vi "Function_Flow Mark.vi"(8 "Error in":errorcluster, 9 "CoordSys In":T1 {"Measurement System"."Axis Reference" items=["Direct", "Indirect"]; "Measurement System"."Angle (deg)" format="%.2f"; "Measurement System"."Origin"."Y" format="%.2f"; "Measurement System"."Origin"."X" format="%.2f"; "Reference System"."Axis Reference" items=["Direct", "Indirect"]; "Reference System"."Angle (deg)" format="%.2f"; "Reference System"."Origin"."Y" format="%.2f"; "Reference System"."Origin"."X" format="%.2f"}, 10 "Data Cluster In":cluster{"Name":string, "Variant In":variant}, 11 "Image Dst In":T4) -> (0 "Error out":errorcluster, 1 "ROI Out":T2 {"Contours"."Type" items=["No Selection", "Point", "Line", "Rectangle", "Oval", "Polygon", "Free", "Annulus", "Unused2", "Unused3", "Broken Line", "Free Hand Line", "Rotated Rectangle"]}, 2 "Result(Flow Mark)":cluster{"Name":string, "NG?":bool, "Score":dbl}, 3 "Objects":T3(array[cluster]) {"Area" format="%.2f"; "Object Center"."Y" format="%.2f"; "Object Center"."X" format="%.2f"}, 4 "Time":u32)   [LabVIEW 2013]
uses:
  <vilib>/vision/Image Controls.llb/IMAQ Image.ctl
  Control/Control_Flow Mark.ctl
  <vilib>/vision/NI_Vision_Development_Module.lvlib
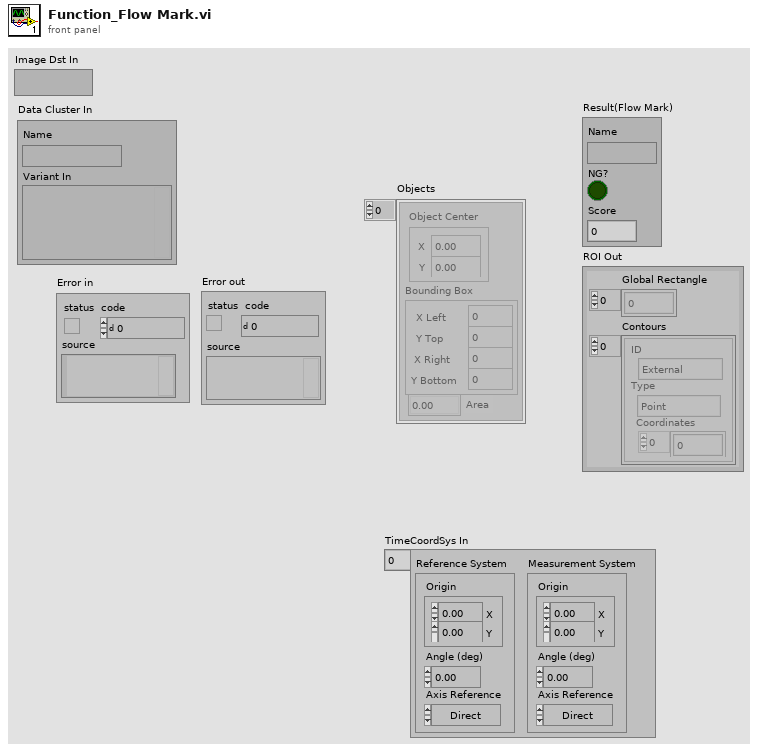
[diagram p1: front panel]
types:
  T1 = typedef "IMAQ Coordinate System" = cluster{"Reference System":cluster{"Origin":cluster{"X":sgl, "Y":sgl}, "Angle (deg)":sgl, "Axis Reference":u32}, "Measurement System":cluster{"Origin":cluster{"X":sgl, "Y":sgl}, "Angle (deg)":sgl, "Axis Reference":u32}}
  T2 = cluster{"Global Rectangle":i32[], "Contours":cluster{"ID":enum32{"External", "Internal"}, "Type":u32, "Coordinates":i32[]}[]}
  T3 = cluster{"Object Center":cluster{"X":dbl, "Y":dbl}, "Bounding Box":cluster{"X Left":dbl, "Y Top":dbl, "X Right":dbl, "Y Bottom":dbl}, "Area":dbl}[]
  T4 = typedef "IMAQ Image.ctl" = refnum<image>
  T5 = typedef "Control_Flow Mark.ctl" = cluster{"Name":string, "ROI":cluster{"Global Rectangle":i32[], "Contours":cluster{"ID":enum32{"External", "Internal"}, "Type":u32, "Coordinates":i32[]}[]}, "Extract Direction(¬y²ª)":enum16{"Left up", "Right up", "Left Down", "Right Down"}, "Extract Potion(¬y²ª)":cluster{"X":i32, "Y":i32}, "Magnification(¬y²ª)":i32, "Settings(¬y²ª)":cluster{"Objects":enum16{"Bright Objects", "Dark Objects"}, "Threshold":i32, "Min Object Size":bool, "Min Size":i32, "Max Object Size":bool, "Max Size":i32}}
  T6 = cluster{"Origin":cluster{"X":sgl, "Y":sgl}, "Angle (deg)":sgl, "Axis Reference":u32}
  T7 = enum16{"Left up", "Right up", "Left Down", "Right Down"}
  T8 = cluster{"Objects":enum16{"Bright Objects", "Dark Objects"}, "Threshold":i32, "Min Object Size":bool, "Min Size":i32, "Max Object Size":bool, "Max Size":i32}
  T9 = typedef "ROI Descriptor" = cluster{"Global Rectangle":i32[], "Contours":cluster{"ID":enum32{"External", "Internal"}, "Type":u32, "Coordinates":i32[]}[]}
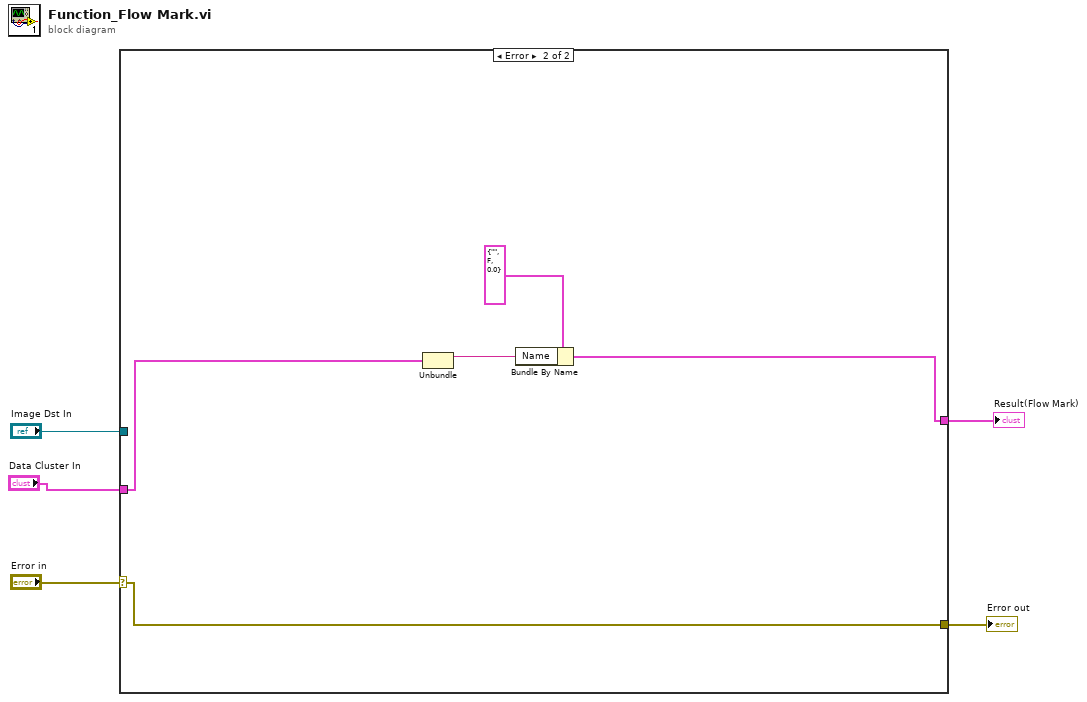
[diagram p0: block diagram]
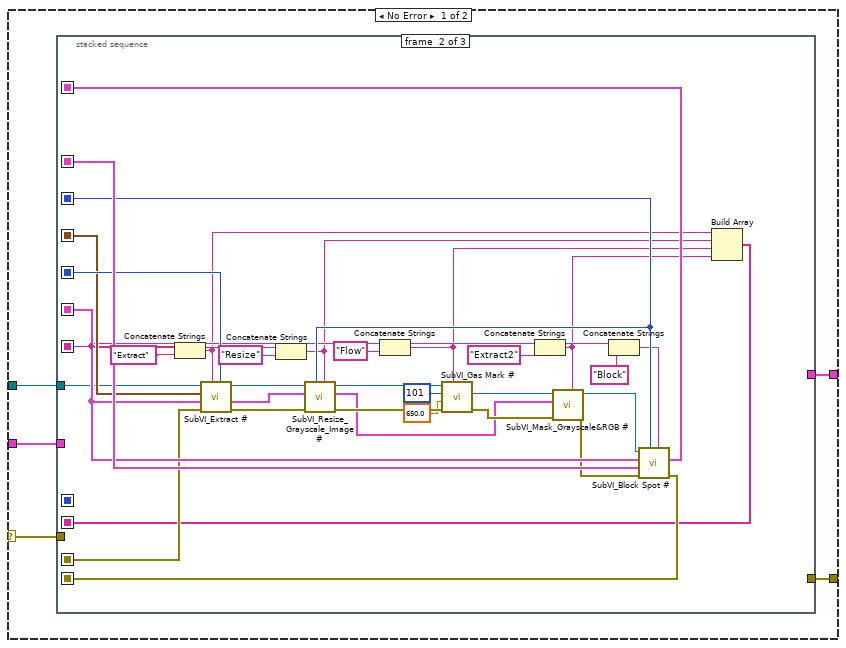
[diagram p2: hidden frame]
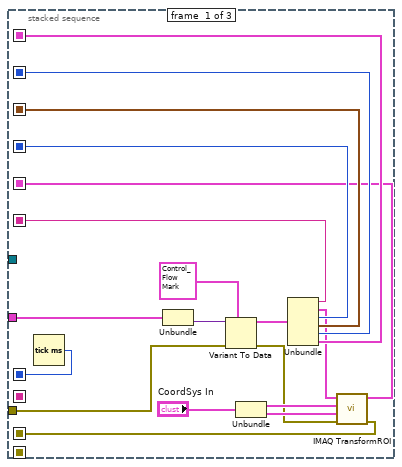
[diagram p3: hidden frame]
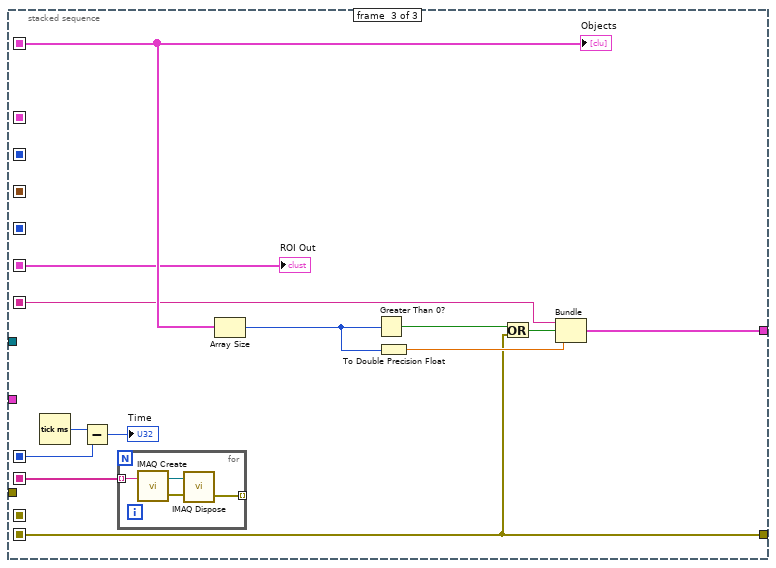
[diagram p4: hidden frame]
diagram:
  n1 = case shown="Error" "Error in" {
    selector: "Error in" -> [w8 w83]
    tunnel: "Image Dst In" -> [w10 _]
    tunnel: [w9 w83] -> w4
    tunnel: [w7 w79] -> w2
    tunnel: "Data Cluster In" -> [w6 w80]
    frame No Error {
      n2 = stacked-sequence {
        seq-local: [w26 _ _] -> [_ w34 w67]
        seq-local: [w15 _ _] -> [_ w50 w64]
        seq-local: [w25 _ _] -> [_ w48 _]
        seq-local: [w24 _ _] -> [_ w47 _]
        seq-local: [w23 _ _] -> [_ w49 _]
        seq-local: [w22 _ _] -> [_ w51 _]
        seq-local: [_ w39 _] -> [_ _ w68]
        seq-local: [_ w38 _] -> [_ _ w66]
        seq-local: [w20 _ _] -> [_ _ w65]
        seq-local: [w12 _ _] -> [_ w37 _]
        seq-local: [_ w29 _] -> [_ _ w63]
        tunnel: w10 -> [_ w46 _]
        tunnel: w8 -> [w14 _ _]
        tunnel: [_ _ w66] -> w9
        tunnel: [_ _ w62] -> w7
        tunnel: w6 -> [w11 _ _]
        frame #0 {
          n3 = Tick Count (ms)() -> (millisecond timer value=w20:u32)
          n4 = Unbundle(w11) -> ("Variant In"=w28:variant)  [unwired: 1 out]
          n5 = Variant To Data(error in=w14, type=T5 {"Name"="", "ROI"={"Global Rectangle"=[], "Contours"=[]}, "Extract Direction(¬y²ª)"=enum."Left up", "Extract Potion(¬y²ª)"={"X"=0, "Y"=0}, "Magnification(¬y²ª)"=2, "Settings(¬y²ª)"={"Objects"=enum."Dark Objects", "Threshold"=100, "Min Object Size"=TRUE, "Min Size"=6, "Max Object Size"=FALSE, "Max Size"=100}} ("¬y²ª_Setting"), Variant=w28) -> (data=w27:T5, error out=w13:errorcluster)
          n6 = Unbundle("CoordSys In") -> ("Reference System"=w18:T6, "Measurement System"=w19:T6)
          n7 = Unbundle(w27) -> ("Name"=w26:string, "ROI"=w16:T2, "Extract Direction(¬y²ª)"=w25:T7, "Extract Potion(¬y²ª)"=w24:cluster{"X":i32, "Y":i32}, "Magnification(¬y²ª)"=w23:i32, "Settings(¬y²ª)"=w22:T8)
          n8 = call "IMAQ TransformROI"("error in (no error)"=w13, "New Reference"=w19, "Base Reference"=w18, "ROI Descriptor"=w16) -> ("error out"=w12:errorcluster, "ROI Descriptor out"=w15:T9)  [unwired: 6 in]
        }
        frame #1 {
          n9 = Concatenate Strings(w34, "Extract" ("Image Register Name")) -> (w33:string)
          n10 = call "SubVI_Extract #.vi"("Extract Direction"=w48, "Image Register Name"=w33, "Error in"=w37, "ROI Descriptor"=w50, "Extract Potion"=w47, "Image Src In"=w46) -> ("Error out"=w59:errorcluster, "ROI Descriptor out"=w40:T9, "Image Dst Out"=w53:T4)  [unwired: 2 in, 1 out]
          n11 = Concatenate Strings(w34, "Resize" ("Image Register Name")) -> (w32:string)
          n12 = call "SubVI_Resize_Grayscale_Image #.vi"("Image Register Name"=w32, "Magnification"=w49, "Error In"=w59, "ROI Descriptor"=w40, "Image Src In"=w53) -> ("Error Out"=w60:errorcluster, "ROI Descriptor out"=w52:T9, "Image Dst Out"=w54:T4)  [unwired: 3 in, 1 out]
          n13 = Concatenate Strings(w34, "Flow" ("Image Register Name")) -> (w31:string)
          n14 = call "SubVI_Gas Mark #.vi"("Image Register Name"=w31, "Error in"=w60, "Divider"=sgl 650.0, "Kernel Size"=101, "Image Src In"=w54) -> ("Error out"=w61:errorcluster, "Image Dst Out"=w55:T4)  [unwired: 4 in, 1 out]
          n15 = Concatenate Strings(w34, "Extract2" ("Image Register Name")) -> (w30:string)
          n16 = call "SubVI_Mask_Grayscale&RGB #.vi"("Image Register Name"=w30, "Error in"=w61, "ROI Descriptor"=w52, "Image Src In"=w55) -> ("Error out"=w45:errorcluster, "Image Dst Out"=w56:T4)  [unwired: 4 in, 2 out]
          n17 = Concatenate Strings(w34, "Block" ("Image Register Name")) -> (w35:string)
          n18 = call "SubVI_Block Spot #.vi"("Image Register Name"=w35, "Magnification"=w49, "Error in"=w45, "Settings"=w51, "ROI Descriptor"=w50, "Image Src In"=w56) -> ("Error out"=w38:errorcluster, "Objects"=w39:T3)  [unwired: 3 in, 1 out]
          n19 = Build Array(w33, w32, w31, w30) -> (w29:string[])
        }
        frame #2 {
          n20 = Tick Count (ms)() -> (millisecond timer value=w73:u32)
          n21 = Subtract(x=w73, y=w65) -> (x-y=→"Time":u32)
          n22 = for {
            tunnel: w63 -> [w78] mode=indexing
            tunnel: [w75] -> _ mode=indexing
            n23 = call "IMAQ Create"("Image Name"=w78) -> ("New Image"=w77:T4, "error out"=w76:errorcluster)  [unwired: 4 in]
            n24 = call "IMAQ Dispose"("Image"=w77, "error in (no error)"=w76) -> ("error out"=w75:errorcluster)  [unwired: 4 in]
          }
          n25 = Array Size(array=w68) -> (size(s)=w69:i32)
          n26 = Greater Than 0?(x=w69) -> (x > 0?=w72:bool)
          n27 = To Double Precision Float(number=w69) -> (double precision float=w70:dbl)
          n28 = Or(x=w72, y=w66) -> (x .or. y?=w71:bool)
          n29 = Bundle("Name"=w67, w71, w70) -> (w62:cluster{"Name":string, bool, dbl})  [unwired: 1 in]
          "Objects" <- w68
          "ROI Out" <- w64
        }
      }
    }
    frame Error {
      n30 = Unbundle(w80) -> ("Name"=w81:string)  [unwired: 1 out]
      n31 = Bundle By Name(cluster=cluster{"Name":string, bool, "Radius":dbl} {"Name"="", FALSE, "Radius"=0.0}, "Name"=w81) -> (w79:cluster{"Name":string, bool, "Radius":dbl})
    }
  }
  "Error out" <- w4
  "Result(Flow Mark)" <- w2
